vi "Predict.vi"(7 "K":i32=5, 9 "Array In":dbl[][](array[numeric]), 10 "Z":dbl, 11 "Y":dbl) -> (0 "Sorted Data points":dbl[][](array[numeric]), 1 "Arrary Out":dbl[][](array[numeric]), 2 "concatenated string":string, 3 "Boolean":bool)   [LabVIEW 2020]
uses:
  7c33d383-65fb-48e9-92ac-9cd8ca6da8bd.vi
  <vilib>/Array/Sort 2D Array - Pop Stack.vi
  <vilib>/Array/Sort 2D Array - Push Stack.vi
  7c33d383-65fb-48e9-92ac-9cd8ca6da8bd.vi/269d4b3b-47f5-49e3-8884-44851e4dd9d5.vi
  7c33d383-65fb-48e9-92ac-9cd8ca6da8bd.vi/6d99389c-673d-4efb-bf33-19b32bcf4cf8.vi
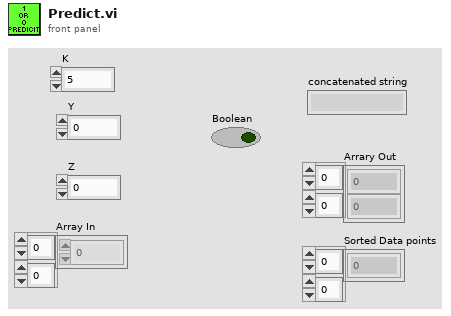
[diagram p1: front panel]
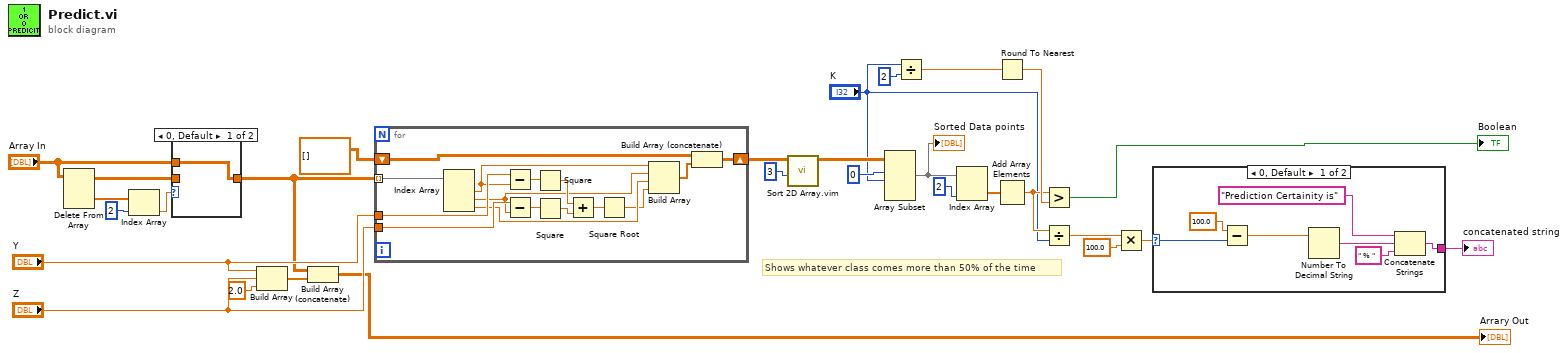
[diagram p0: block diagram]
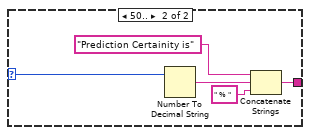
[diagram p2: hidden frame]
diagram:
  # "Shows whatever class comes more than 50% of the time"
  n1 = Delete From Array(array="Array In") -> (deleted portion=w12:dbl[], array with subset deleted=w8:dbl[][])  [unwired: 3 in]
  n2 = Index Array(array=w12, index=2) -> (element=w10:dbl)
  n3 = case shown="0, Default" w10 {
    tunnel: "Array In" -> [w30 _]
    tunnel: w8 -> [_ w31]
    tunnel: [w30 w31] -> w7
    frame 0, Default {
    }
    frame 2 {
    }
  }
  n4 = Build Array("Y", "Z", 2.0 ("element")) -> (w14:dbl[])
  n5 = Build Array (concatenate)(w7, w14) -> (→"Arrary Out":dbl[][])
  n6 = for {
    tunnel: w7 -> [w46] mode=indexing
    tunnel: "Y" -> [w45]
    tunnel: "Z" -> [w44]
    shift-right: [w36] -> w22
    shift-left: dbl[][] [] -> [w37]
    n7 = Index Array(array=w46) -> (element #1=w35:dbl, element #2=w34:dbl, element #3=w33:dbl)  [unwired: 3 in]
    n8 = Subtract(x=w45, y=w35) -> (x-y=w43:dbl)
    n9 = Subtract(x=w44, y=w34) -> (x-y=w42:dbl)
    n10 = Square(x=w43) -> (x^2=w41:dbl)
    n11 = Square(x=w42) -> (x^2=w40:dbl)
    n12 = Add(x=w41, y=w40) -> (x+y=w39:dbl)
    n13 = Square Root(x=w39) -> (sqrt(x)=w32:dbl)
    n14 = Build Array(w35, w34, w33, w32) -> (w38:dbl[])
    n15 = Build Array (concatenate)(w37, w38) -> (w36:dbl[][])
  }
  n16 = call "Sort 2D Array.vim"("index"=3, "2D array"=w22) -> ("sorted 2D array"=w24:dbl[][])  [unwired: 8 in, 1 out]
  n17 = Array Subset(array=w24, index (row)=0 ("index"), length (row)="K") -> (w26:dbl[][])  [unwired: 2 in]
  "Sorted Data points" <- w26
  n18 = Divide(x="K", y=2) -> (x/y=w19:dbl)
  n19 = Index Array(array=w26, index (col)=2 ("disabled index (col)")) -> (element=w28:dbl[])  [unwired: 1 in]
  n20 = Round To Nearest(number=w19) -> (nearest integer value=w18:dbl)
  n21 = Add Array Elements(numeric array=w28) -> (sum=w6:dbl)
  n22 = Greater?(x=w6, y=w18) -> (0:→"Boolean":bool)
  n23 = Divide(x=w6, y="K") -> (x/y=w4:dbl)
  n24 = Multiply(x=w4, y=100.0) -> (x*y=w2:dbl)
  n25 = case shown="0, Default" w2 {
    selector: w2 -> [w48 w58]
    tunnel: [w50 w54] -> w1
    frame 0, Default {
      n26 = Subtract(x=100.0, y=w48) -> (x-y=w47:dbl)
      n27 = Number To Decimal String(number=w47) -> (decimal integer string=w53:string)  [unwired: 1 in]
      n28 = Concatenate Strings("Prediction Certainity is" ("string"), w53, " % ") -> (w50:string)
    }
    frame 50.. {
      n29 = Number To Decimal String(number=w58) -> (decimal integer string=w57:string)  [unwired: 1 in]
      n30 = Concatenate Strings("Prediction Certainity is" ("string"), w57, " % ") -> (w54:string)
    }
  }
  "concatenated string" <- w1
